vi "Config-Get Sections.vi"(0 "configuration file path":path, 11 "error in (no error)":errorcluster) -> (4 "file path":path, 8 "section names":string[](array[string]), 15 "error out":errorcluster)   [LabVIEW 2020]
uses:
  <vilib>/Utility/config.llb/NI_LVConfig.lvlib
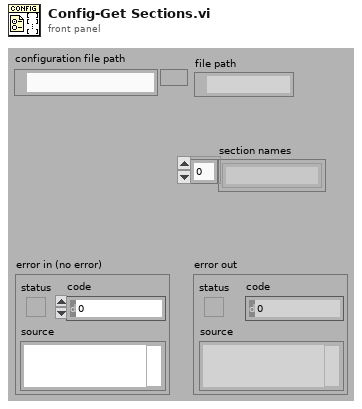
[diagram p1: front panel]
types:
  T1 = typedef "NI_LVConfig.lvlib/Config Data RefNum.ctl" = refnum<k1>
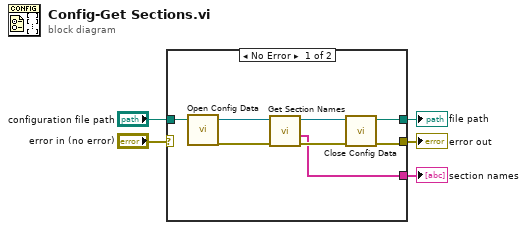
[diagram p0: block diagram]
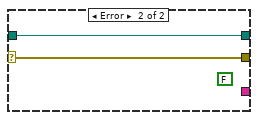
[diagram p2: hidden frame]
diagram:
  n1 = case shown="No Error" "error in (no error)" {
    selector: "error in (no error)" -> [_ w15]
    tunnel: [w11 w15] -> w5
    tunnel: "configuration file path" -> [w8 w14]
    tunnel: [w7 w14] -> w2
    tunnel: [w6 _] -> w1
    frame No Error {
      n2 = call <vilib>:"Open Config Data.vi"("configuration file path"=w8) -> ("error out"=w13:errorcluster, "refnum"=w12:T1)  [unwired: 8 in, 1 out]
      n3 = call <vilib>:"Get Section Names.vi"("error in (no error)"=w13, "refnum"=w12) -> ("error out"=w10:errorcluster, "section names"=w6:string[], "refnum out"=w9:T1)  [unwired: 7 in]
      n4 = call <vilib>:"Close Config Data.vi"("error in (no error)"=w10, "refnum"=w9) -> ("error out"=w11:errorcluster, "file path"=w7:path)  [unwired: 8 in]
    }
    frame Error {
      (unwired) FALSE ("found?")
    }
  }
  "error out" <- w5
  "file path" <- w2
  "section names" <- w1
